vi "tsc--Color Picker.vi"(6 "VI Position":cluster{"Left":i16, "Top":i16}={"Left"=-1, "Top"=-1}, 11 "input":u32(colorbox)) -> (2 "accepted?":bool, 3 "Resolved Color":u32(colorbox))   [LabVIEW 2021, in "Material SubVIs.lvlib"]
doc: "Allow user to pick a color by slider bar entry for RGB values and/or by HEX code entry. See preview of resolved color before accepting or cancelling.\n\n<b>Code Developed By:</b> +\nDaniel Coons +\nTechnology Service Corporation +\nwww.tsc.com/atcs"
uses:
  Material SubVIs.lvlib
  <vilib>/Utility/miscctls.llb/LVRectTypeDef.ctl
  <vilib>/UserTags/UserTags.lvlib
panel:
  in  "HSL":bool
  in  "RGB":bool
  in  "Tab Control":enum32{"rgb", "hsl"}(tab)
  in  "R-number":u8(slide) scale=0.0..255.0
  in  "G-number":u8(slide) scale=0.0..255.0
  in  "B-number":u8(slide) scale=0.0..255.0
  out "R":u32[](array[colorbox])
  out "G":u32[](array[colorbox])
  out "B":u32[](array[colorbox])
  in  "R-selector":u8
  in  "G-selector":u8
  in  "B-selector":u8
  in  "H-number":u16(slide) max=360 scale=0.0..360.0
  in  "S-number":u8(slide) max=100 scale=0.0..100.0
  in  "L-number":u8(slide) max=100 scale=0.0..100.0
  out "S":u32[](array[colorbox])
  out "L":u32[](array[colorbox])
  in  "H-selector":u16 max=360
  in  "S-selector":u8 max=100
  in  "L-selector":u8 max=100
  out "H":u32[](array[colorbox])
  in  "cancel":bool
  in  "ok":bool
  in  "Hex Color":u32 max=16777215 format="%06x"
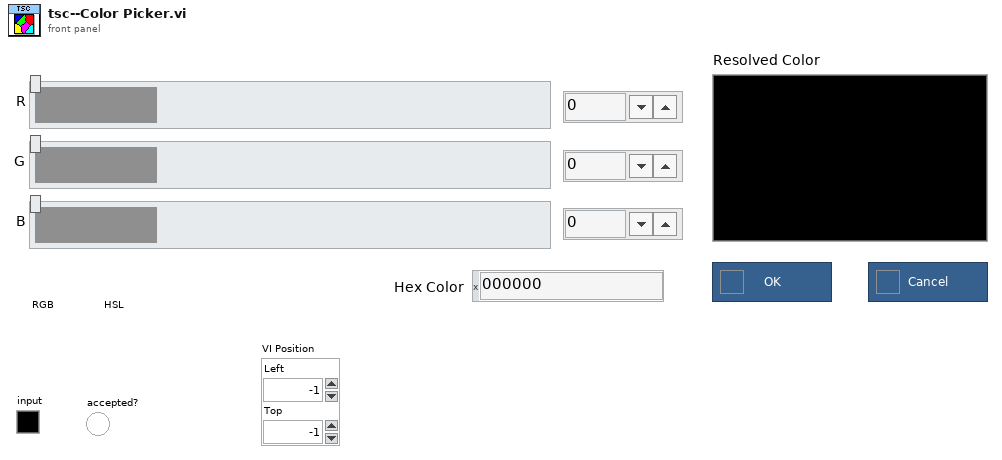
[diagram p1: front panel]
types:
  T1 = typedef "LVRectTypeDef.ctl" = cluster{"Left":i16, "Top":i16, "Right":i16, "Bottom":i16}
  T2 = typedef "LVPointTypeDef.ctl" = cluster{"Horizontal":i16, "Vertical":i16}
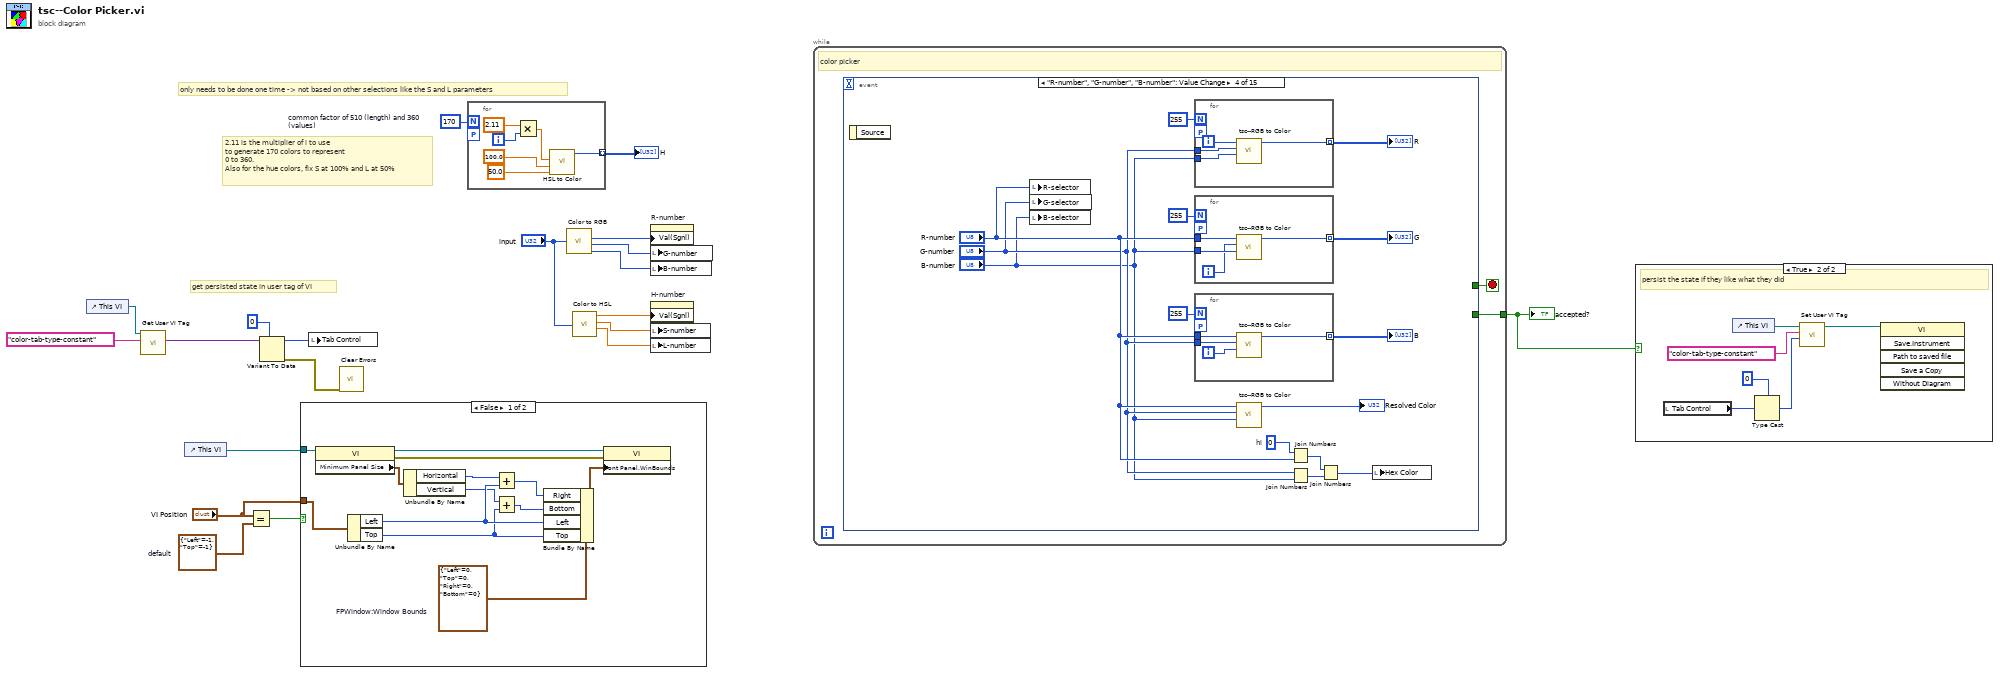
[diagram p0: block diagram]
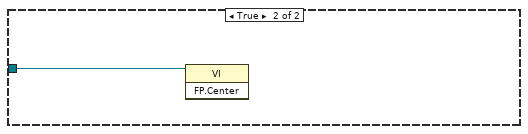
[diagram p3: hidden frame]
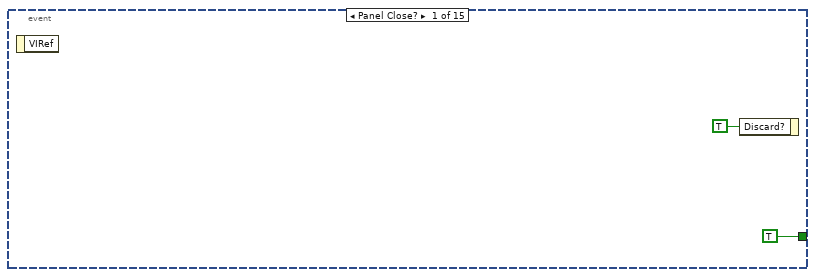
[diagram p4: hidden frame]
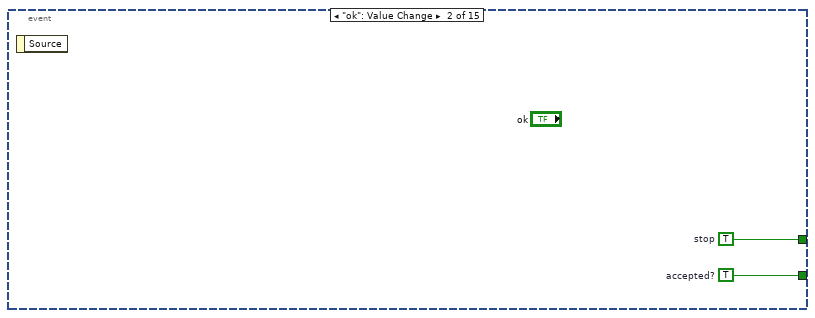
[diagram p5: hidden frame]
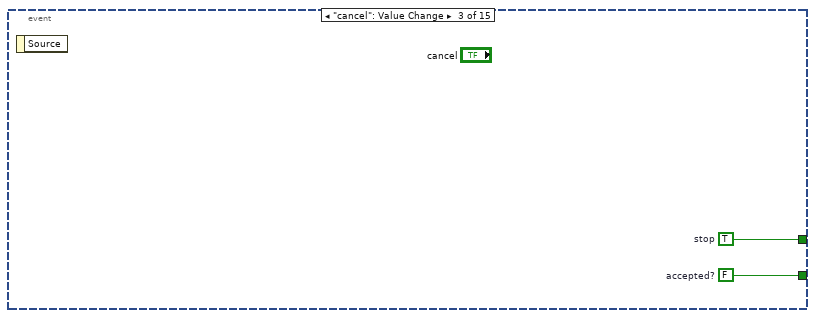
[diagram p6: hidden frame]
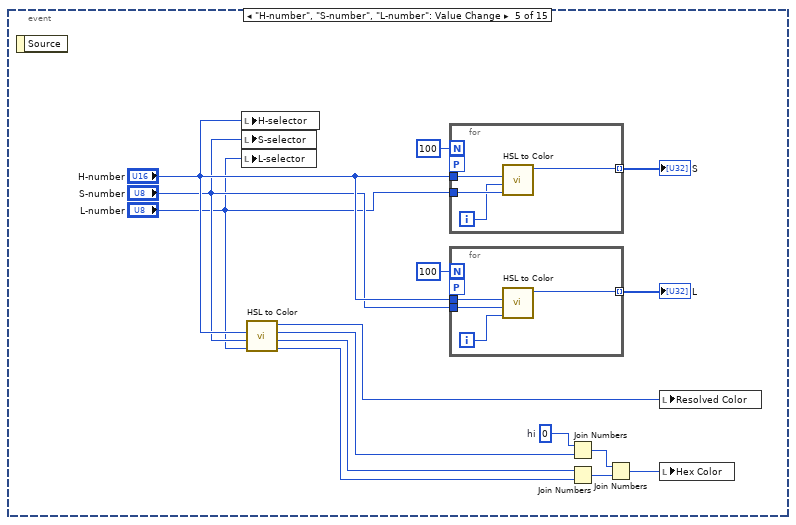
[diagram p7: hidden frame]
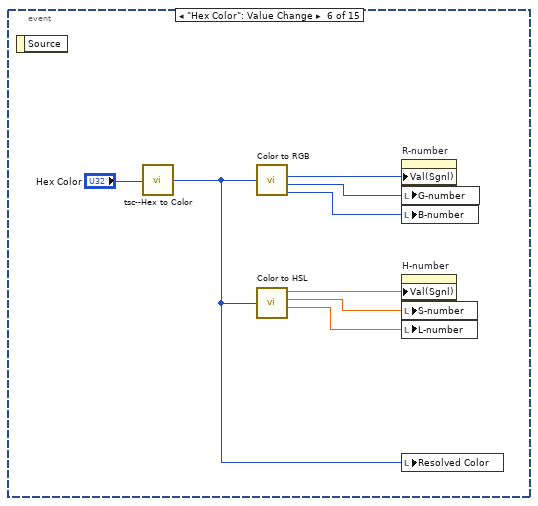
[diagram p8: hidden frame]
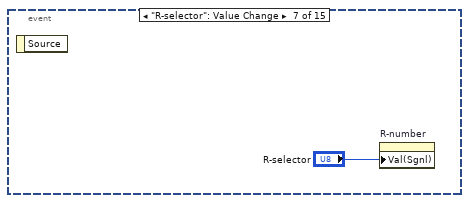
[diagram p9: hidden frame]
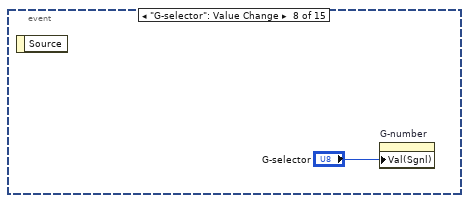
[diagram p10: hidden frame]
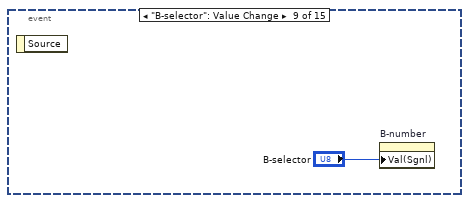
[diagram p11: hidden frame]
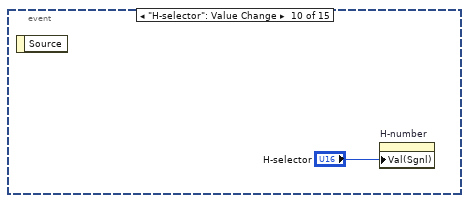
[diagram p12: hidden frame]
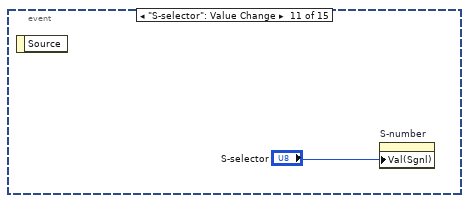
[diagram p13: hidden frame]
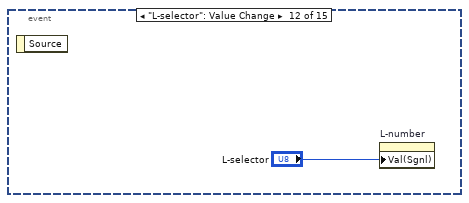
[diagram p14: hidden frame]
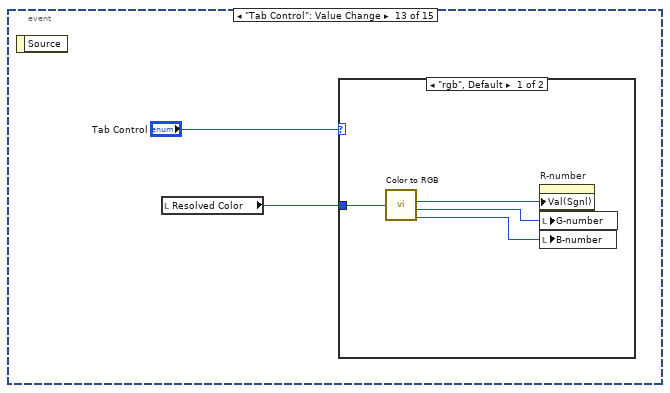
[diagram p15: hidden frame]
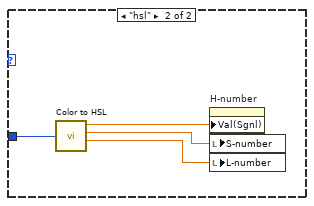
[diagram p16: hidden frame]
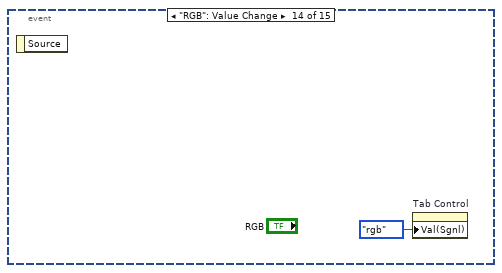
[diagram p17: hidden frame]
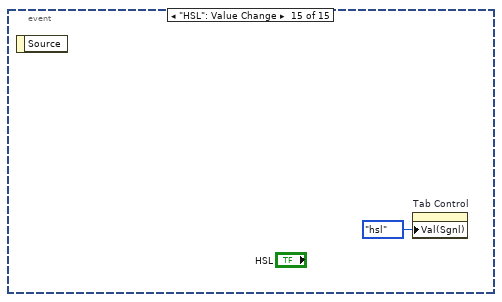
[diagram p18: hidden frame]
diagram:
  w8 = 170  # common factor of 510 (length) and 360 (values)
  w16 = cluster{"Left":i16, "Top":i16} {"Left"=-1, "Top"=-1}  # default
  # "get persisted state in user tag of VI"
  # "only needs to be done one time -> not based on other selections like the S and L parameters"
  # "2.11 is the multiplier of i to use\nto generate 170 colors to represent\n0 to 360. \nAlso for the hue colors, fix S at 100% and L at 50%"
  n1 = control-ref of="This VI"() -> (w7:refnum<vi>)
  n2 = call <vilib>:"Get User VI Tag.vi"("Tag Name"="color-tab-type-constant", "VI Refnum"=w7) -> ("Value"=w5:variant)  [unwired: 6 in, 3 out]
  n3 = control-ref of="This VI"() -> (w17:refnum<vi>)
  n4 = Equal?(x="VI Position", y=w16) -> (x = y?=w15:bool)
  n5 = Variant To Data(type=u32 0, Variant=w5) -> (data=w4:u32, error out=w2:errorcluster)  [unwired: 1 in]
  n6 = case shown="False" w15 {
    tunnel: w17 -> [w33 w34]
    tunnel: "VI Position" -> [w29 _]
    frame False {
      w28 = T1 {"Left"=0, "Top"=0, "Right"=0, "Bottom"=0}  # FPWindow:Window Bounds
      n7 = property class="VI"(reference=w33) -> (reference out=w32:refnum<vi>, error out=w31:errorcluster, "Minimum Panel Size"=w30:T2)  [unwired: 1 in]
      n8 = Unbundle By Name(w29) -> ("Left"=w27:i16, "Top"=w22:i16)
      n9 = Unbundle By Name(w30) -> ("Horizontal"=w26:i16, "Vertical"=w23:i16)
      n10 = Add(x=w26, y=w27) -> (x+y=w25:i16)
      n11 = Add(x=w23, y=w22) -> (x+y=w21:i16)
      n12 = Bundle By Name(cluster=w28, "Right"=w25, "Bottom"=w21, "Left"=w27, "Top"=w22) -> (w24:T1)
      n13 = property class="VI"(reference=w32, error in=w31, "Front Panel.WinBounds"=w24) -> ()  [unwired: 2 out]
    }
    frame True {
      n14 = invoke class="VI" method="FP.Center"(reference=w34) -> ()  [unwired: 2 in, 3 out]
    }
  }
  n15 = local write "Tab Control"(w4) -> ()
  n16 = call <vilib>:"Clear Errors.vi"("error in (no error)"=w2) -> ()  [unwired: 5 in, 2 out]
  n17 = for {
    N: w8 -> [_]
    tunnel: [w40] -> w9 mode=indexing
    workers-P: _ -> [_]
    i -> [w36]
    n18 = Multiply(x=2.11, y=w36) -> (x*y=w35:dbl)
    n19 = call "HSL to Color.vi"("L (%)"=50.0, "S (%)"=100.0, "H (degrees)"=w35) -> ("Color out"=w40:u32)  [unwired: 5 in, 3 out]
  }
  "H" <- w9
  n20 = call <vilib>:"Color to RGB.vi"("Color"="input") -> ("R"=w20:u8, "G"=w19:u8, "B"=w18:u8)  [unwired: 1 out]
  n21 = call "Color to HSL.vi"("Color In"="input") -> ("H (degrees)"=w10:dbl, "S (%)"=w11:dbl, "L (%)"=w12:dbl)  [unwired: 4 in, 1 out]
  n22 = property on="R-number" class="Slide (strict)"("Val(Sgnl)"=w20) -> ()  [unwired: 2 in, 2 out]
  n23 = local write "G-number"(w19) -> ()
  n24 = local write "B-number"(w18) -> ()
  n25 = property on="H-number" class="Slide (strict)"("Val(Sgnl)"=w10) -> ()  [unwired: 2 in, 2 out]
  n26 = local write "S-number"(w11) -> ()
  n27 = local write "L-number"(w12) -> ()
  n28 = while {
    tunnel: [w41] -> w1
    stop <- w42 stop-if-true
    # "color picker"
    n29 = event shown="[3] \"R-number\", \"G-number\", \"B-number\": Value Change" {
      selector: _ -> [_ _ _ _ _ _ _ _ _ _ _ _ _ _ _]
      dyn-events: _ -> [_ _ _ _ _ _ _ _ _ _ _ _ _ _ _]
      timeout: _ -> [_ _ _ _ _ _ _ _ _ _ _ _ _ _ _]
      tunnel: [TRUE w46 w48 _ _ _ _ _ _ _ _ _ _ _ _] -> w42
      tunnel: [_ w45 w47 _ _ _ _ _ _ _ _ _ _ _ _] -> w41
      event Panel Close? {
        n30 = event-data() -> ()  [unwired: 1 in, 1 out]
        n31 = event-data("Discard?"=TRUE) -> ()  [unwired: 1 in, 1 out]
      }
      event "ok": Value Change {
        w45 = TRUE  # accepted?
        w46 = TRUE  # stop
        n32 = event-data() -> ()  [unwired: 1 in, 1 out]
      }
      event "cancel": Value Change {
        w47 = FALSE  # accepted?
        w48 = TRUE  # stop
        n33 = event-data() -> ()  [unwired: 1 in, 1 out]
      }
      event "R-number", "G-number", "B-number": Value Change {
        w56 = u8 0  # hi
        n34 = event-data() -> ()  [unwired: 1 in, 1 out]
        n35 = local write "R-selector"("R-number") -> ()
        n36 = local write "G-selector"("G-number") -> ()
        n37 = local write "B-selector"("B-number") -> ()
        n38 = for {
          N: 255 -> [_]
          tunnel: "G-number" -> [w74]
          tunnel: "B-number" -> [w73]
          tunnel: [w71] -> w61 mode=indexing
          workers-P: _ -> [_]
          i -> [w72]
          n39 = call "tsc--RGB to Color.vi"("B"=w73, "G"=w74, "R"=w72) -> ("Color"=w71:u32)  [unwired: 8 in]
        }
        "R" <- w61
        n40 = for {
          N: 255 -> [_]
          tunnel: "B-number" -> [w70]
          tunnel: [w69] -> w58 mode=indexing
          tunnel: "R-number" -> [w67]
          workers-P: _ -> [_]
          i -> [w68]
          n41 = call "tsc--RGB to Color.vi"("B"=w70, "G"=w68, "R"=w67) -> ("Color"=w69:u32)  [unwired: 8 in]
        }
        "G" <- w58
        n42 = for {
          N: 255 -> [_]
          tunnel: "R-number" -> [w64]
          tunnel: [w66] -> w57 mode=indexing
          tunnel: "G-number" -> [w63]
          workers-P: _ -> [_]
          i -> [w65]
          n43 = call "tsc--RGB to Color.vi"("B"=w65, "G"=w63, "R"=w64) -> ("Color"=w66:u32)  [unwired: 8 in]
        }
        "B" <- w57
        n44 = call "tsc--RGB to Color.vi"("B"="B-number", "G"="G-number", "R"="R-number") -> ("Color"=→"Resolved Color":u32)  [unwired: 8 in]
        n45 = Join Numbers(hi=w56, lo="R-number") -> ((hi.lo)=w54:u16)
        n46 = Join Numbers(hi="G-number", lo="B-number") -> ((hi.lo)=w55:u16)
        n47 = Join Numbers(hi=w54, lo=w55) -> ((hi.lo)=w53:u32)
        n48 = local write "Hex Color"(w53) -> ()
      }
      event "H-number", "S-number", "L-number": Value Change {
        w87 = u8 0  # hi
        n49 = event-data() -> ()  [unwired: 1 in, 1 out]
        n50 = local write "H-selector"("H-number") -> ()
        n51 = local write "S-selector"("S-number") -> ()
        n52 = local write "L-selector"("L-number") -> ()
        n53 = call "HSL to Color.vi"("L (%)"="L-number", "S (%)"="S-number", "H (degrees)"="H-number") -> ("B"=w76:u8, "G"=w78:u8, "R"=w80:u8, "Color out"=w75:u32)  [unwired: 5 in]
        n54 = for {
          N: 100 -> [_]
          tunnel: "L-number" -> [w97]
          tunnel: [w96] -> w83 mode=indexing
          tunnel: "H-number" -> [w94]
          workers-P: _ -> [_]
          i -> [w95]
          n55 = call "HSL to Color.vi"("L (%)"=w97, "S (%)"=w95, "H (degrees)"=w94) -> ("Color out"=w96:u32)  [unwired: 5 in, 3 out]
        }
        "S" <- w83
        n56 = for {
          N: 100 -> [_]
          tunnel: "H-number" -> [w91]
          tunnel: [w93] -> w82 mode=indexing
          tunnel: "S-number" -> [w90]
          workers-P: _ -> [_]
          i -> [w92]
          n57 = call "HSL to Color.vi"("L (%)"=w92, "S (%)"=w90, "H (degrees)"=w91) -> ("Color out"=w93:u32)  [unwired: 5 in, 3 out]
        }
        "L" <- w82
        n58 = Join Numbers(hi=w87, lo=w80) -> ((hi.lo)=w85:u16)
        n59 = Join Numbers(hi=w78, lo=w76) -> ((hi.lo)=w86:u16)
        n60 = Join Numbers(hi=w85, lo=w86) -> ((hi.lo)=w84:u32)
        n61 = local write "Resolved Color"(w75) -> ()
        n62 = local write "Hex Color"(w84) -> ()
      }
      event "Hex Color": Value Change {
        n63 = event-data() -> ()  [unwired: 1 in, 1 out]
        n64 = call "tsc--Hex to Color.vi"("Hex String"="Hex Color") -> ("Color"=w99:u32)  [unwired: 4 in]
        n65 = call <vilib>:"Color to RGB.vi"("Color"=w99) -> ("R"=w102:u8, "G"=w101:u8, "B"=w100:u8)  [unwired: 1 out]
        n66 = call "Color to HSL.vi"("Color In"=w99) -> ("H (degrees)"=w104:dbl, "S (%)"=w103:dbl, "L (%)"=w98:dbl)  [unwired: 4 in, 1 out]
        n67 = property on="R-number" class="Slide (strict)"("Val(Sgnl)"=w102) -> ()  [unwired: 2 in, 2 out]
        n68 = local write "G-number"(w101) -> ()
        n69 = local write "B-number"(w100) -> ()
        n70 = property on="H-number" class="Slide (strict)"("Val(Sgnl)"=w104) -> ()  [unwired: 2 in, 2 out]
        n71 = local write "S-number"(w103) -> ()
        n72 = local write "L-number"(w98) -> ()
        n73 = local write "Resolved Color"(w99) -> ()
      }
      event "R-selector": Value Change {
        n74 = event-data() -> ()  [unwired: 1 in, 1 out]
        n75 = property on="R-number" class="Slide (strict)"("Val(Sgnl)"="R-selector") -> ()  [unwired: 2 in, 2 out]
      }
      event "G-selector": Value Change {
        n76 = event-data() -> ()  [unwired: 1 in, 1 out]
        n77 = property on="G-number" class="Slide (strict)"("Val(Sgnl)"="G-selector") -> ()  [unwired: 2 in, 2 out]
      }
      event "B-selector": Value Change {
        n78 = event-data() -> ()  [unwired: 1 in, 1 out]
        n79 = property on="B-number" class="Slide (strict)"("Val(Sgnl)"="B-selector") -> ()  [unwired: 2 in, 2 out]
      }
      event "H-selector": Value Change {
        n80 = event-data() -> ()  [unwired: 1 in, 1 out]
        n81 = property on="H-number" class="Slide (strict)"("Val(Sgnl)"="H-selector") -> ()  [unwired: 2 in, 2 out]
      }
      event "S-selector": Value Change {
        n82 = event-data() -> ()  [unwired: 1 in, 1 out]
        n83 = property on="S-number" class="Slide (strict)"("Val(Sgnl)"="S-selector") -> ()  [unwired: 2 in, 2 out]
      }
      event "L-selector": Value Change {
        n84 = event-data() -> ()  [unwired: 1 in, 1 out]
        n85 = property on="L-number" class="Slide (strict)"("Val(Sgnl)"="L-selector") -> ()  [unwired: 2 in, 2 out]
      }
      event "Tab Control": Value Change {
        n86 = event-data() -> ()  [unwired: 1 in, 1 out]
        n87 = local read "Resolved Color"() -> (w112:u32)
        n88 = case shown="\"rgb\", Default" "Tab Control" {
          tunnel: w112 -> [w117 w121]
          frame "rgb", Default {
            n89 = call <vilib>:"Color to RGB.vi"("Color"=w117) -> ("R"=w116:u8, "G"=w115:u8, "B"=w114:u8)  [unwired: 1 out]
            n90 = property on="R-number" class="Slide (strict)"("Val(Sgnl)"=w116) -> ()  [unwired: 2 in, 2 out]
            n91 = local write "G-number"(w115) -> ()
            n92 = local write "B-number"(w114) -> ()
          }
          frame "hsl" {
            n93 = call "Color to HSL.vi"("Color In"=w121) -> ("H (degrees)"=w120:dbl, "S (%)"=w119:dbl, "L (%)"=w118:dbl)  [unwired: 4 in, 1 out]
            n94 = property on="H-number" class="Slide (strict)"("Val(Sgnl)"=w120) -> ()  [unwired: 2 in, 2 out]
            n95 = local write "S-number"(w119) -> ()
            n96 = local write "L-number"(w118) -> ()
          }
        }
      }
      event "RGB": Value Change {
        n97 = event-data() -> ()  [unwired: 1 in, 1 out]
        n98 = property on="Tab Control" class="TabCtl (strict)"("Val(Sgnl)"=enum32{"rgb", "hsl"}."rgb" ("Value (Signaling)")) -> ()  [unwired: 2 in, 2 out]
      }
      event "HSL": Value Change {
        n99 = event-data() -> ()  [unwired: 1 in, 1 out]
        n100 = property on="Tab Control" class="TabCtl (strict)"("Val(Sgnl)"=enum32{"rgb", "hsl"}."hsl" ("Value (Signaling)")) -> ()  [unwired: 2 in, 2 out]
      }
    }
  }
  "accepted?" <- w1
  n101 = case shown="True" w1 {
    frame False {
    }
    frame True {
      # "persist the state if they like what they did"
      n102 = local read "Tab Control"() -> (w129:enum32{"rgb", "hsl"})
      n103 = control-ref of="This VI"() -> (w127:refnum<vi>)
      n104 = Type Cast(type=u32 0, x=w129) -> (*(type *) &x=w125:u32)
      n105 = call <vilib>:"Set User VI Tag.vi"("Value"=w125, "Tag Name"="color-tab-type-constant", "VI Refnum"=w127) -> ("dup VI Refnum"=w124:refnum<vi>)  [unwired: 6 in, 2 out]
      n106 = invoke class="VI" method="Save.Instrument"(reference=w124) -> ()  [unwired: 5 in, 6 out]
    }
  }
